vi "Generate step array.vi"(4 "Step":dbl, 6 "Add step back":bool, 7 "Increment mode":T1, 9 "Number of steps":i32, 10 "End":dbl, 11 "Start":dbl) -> (3 "Steps":dbl[](array[numeric]))   [LabVIEW 2019]
uses:
  Increment mode.ctl
panel:
  out "Steps graph":dbl[](graph)
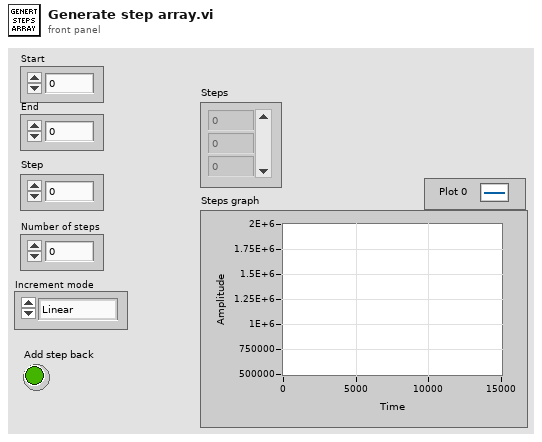
[diagram p1: front panel]
types:
  T1 = typedef "Increment mode.ctl" = enum16{"Linear", "Square root", "Square", "Log", "Exponent"}
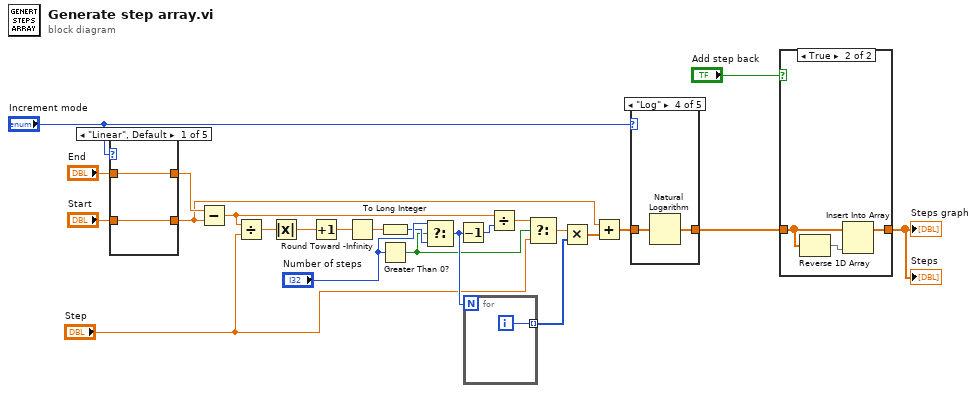
[diagram p0: block diagram]
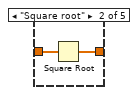
[diagram p4: hidden frame]
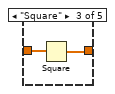
[diagram p5: hidden frame]
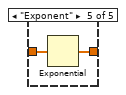
[diagram p6: hidden frame]
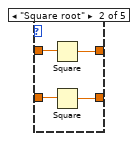
[diagram p7: hidden frame]
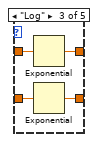
[diagram p8: hidden frame]
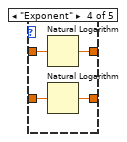
[diagram p9: hidden frame]
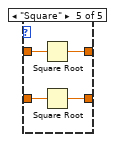
[diagram p10: hidden frame]
diagram:
  n1 = case shown="\"Linear\", Default" "Increment mode" {
    tunnel: [w26 w30 w34 w38 w42] -> w24
    tunnel: "End" -> [w26 w29 w33 w37 w41]
    tunnel: "Start" -> [w25 w28 w32 w36 w40]
    tunnel: [w25 w27 w31 w35 w39] -> w2
    frame "Linear", Default {
    }
    frame "Square root" {
      n2 = Square(x=w29) -> (x^2=w30:dbl)
      n3 = Square(x=w28) -> (x^2=w27:dbl)
    }
    frame "Log" {
      n4 = Exponential(1:w33) -> (0:w34:dbl)
      n5 = Exponential(1:w32) -> (0:w31:dbl)
    }
    frame "Exponent" {
      n6 = Natural Logarithm(1:w37) -> (0:w38:dbl)
      n7 = Natural Logarithm(1:w36) -> (0:w35:dbl)
    }
    frame "Square" {
      n8 = Square Root(x=w41) -> (sqrt(x)=w42:dbl)
      n9 = Square Root(x=w40) -> (sqrt(x)=w39:dbl)
    }
  }
  n10 = Subtract(x=w24, y=w2) -> (x-y=w10:dbl)
  n11 = Divide(x=w10, y="Step") -> (x/y=w11:dbl)
  n12 = Absolute Value(x=w11) -> (abs(x)=w14:dbl)
  n13 = Increment(x=w14) -> (x+1=w12:dbl)
  n14 = Round Toward -Infinity(1:w12) -> (0:w13:dbl)
  n15 = To Long Integer(number=w13) -> (32bit integer=w9:i32)
  n16 = Greater Than 0?(x="Number of steps") -> (x > 0?=w8:bool)
  n17 = Select(t="Number of steps", s=w8, f=w9) -> (s? t:f=w15:i32)
  n18 = Decrement(x=w15) -> (x-1=w21:i32)
  n19 = for {
    N: w15 -> [_]
    tunnel: [w43] -> w3 mode=indexing
    i -> [w43]
  }
  n20 = Divide(x=w10, y=w21) -> (x/y=w7:dbl)
  n21 = Select(t=w7, s=w8, f="Step") -> (s? t:f=w4:dbl)
  n22 = Multiply(x=w4, y=w3) -> (x*y=w5:dbl[])
  n23 = Add(x=w2, y=w5) -> (x+y=w1:dbl[])
  n24 = case shown="\"Log\"" "Increment mode" {
    tunnel: w1 -> [w44 w46 w48 w50 w52]
    tunnel: [w44 w45 w47 w49 w51] -> w19
    frame "Linear", Default {
    }
    frame "Square root" {
      n25 = Square Root(x=w46) -> (sqrt(x)=w45:dbl[])
    }
    frame "Square" {
      n26 = Square(x=w48) -> (x^2=w47:dbl[])
    }
    frame "Log" {
      n27 = Natural Logarithm(1:w50) -> (0:w49:dbl[])
    }
    frame "Exponent" {
      n28 = Exponential(1:w52) -> (0:w51:dbl[])
    }
  }
  n29 = case shown="True" "Add step back" {
    tunnel: w19 -> [w53 w56]
    tunnel: [w53 w54] -> w18
    frame False {
    }
    frame True {
      n30 = Reverse 1D Array(array=w56) -> (reversed array=w55:dbl[])
      n31 = Insert Into Array(array=w56, new element=w55) -> (w54:dbl[])  [unwired: 1 in]
    }
  }
  "Steps" <- w18
  "Steps graph" <- w18
